vi "svx_Polar_Add_Task.vi"(9 "task list":T1[](array[typedef]), 10 "new task":T1) -> (2 "task list out":T1[](array[typedef]))   [LabVIEW 2017, in "SVX Polar Plot.xctl"]
uses:
  <vilib>/addons/_XControls/Polar Plot/SVX Polar Plot.xctl
  <vilib>/addons/_XControls/Polar Plot/subVIs/svx_Polar_Exe_Tasks.ctl
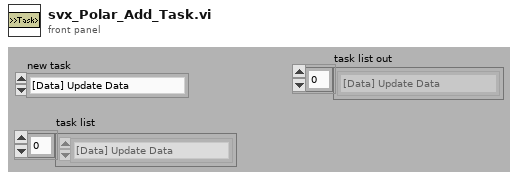
[diagram p1: front panel]
types:
  T1 = typedef "SVX Polar Plot.xctl/svx_Polar_Exe_Tasks.ctl" = enum16{"[Data] Update Data", "[Scale] Update Polar Scale", "[Scale] Autoscale", "[Legend] Update Legend", "[Cursor] Cursor Release", "[Pane] Change Minimum Size", "[Annt] Upodate Annotation", "[Plot] Appearance", "[Cursor] Visibility", "[Cursor] Appearance", "[Cursor] Index", "[Scale] MagnitudeVisibility", "[Scale] PhaseVisibility", "[Scale] PhaseAppearance", "[Scale] MagnitudeApperance", "[Plot] AcceptanceRegion", "[Scale] RangeChange", "[Marker] Appearance", "[Marker] List", "[Marker] Visibility", "[Legend] Visibility", "[Legend] Color", "[Data] Index", "[Legend] Update String", "[Cursor] Trigger Event", "[Scale] Trigger Event", "[Data] Clear Graph"}
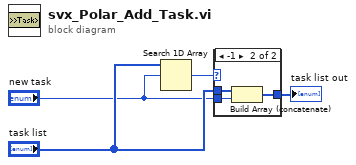
[diagram p0: block diagram]
diagram:
  n1 = Search 1D Array(1D array="task list", element="new task") -> (index of element=w4:i32)  [unwired: 1 in]
  n2 = case shown="-1" w4 {
    tunnel: [w5 w8] -> w1
    tunnel: "task list" -> [w5 w7]
    tunnel: "new task" -> [_ w6]
    frame 0, Default {
    }
    frame -1 {
      n3 = Build Array (concatenate)(w7, w6) -> (w8:T1[])
    }
  }
  "task list out" <- w1
